vi "GV_FindEqualUnits.vi"(11 "TAGproperties":T1=[{"TAG"="ch0001", "Qtype"="PAQ", "TAGprop"={"Description"="", "EngUnits"="", "RangeH"=-1.0, "RangeL"=-1.0, "Resolution"=-1, "Obsolete"=FALSE, "ChangeDate"=timestamp(3692433115.085 s since 1904-01-01), "ChangeSource"="AVPP", "ChangeReason"="100 Unidentified TAGs sent by HISW", "TagFunc"=0}}, {"TAG"="ch0002", "Qtype"="PAQ", "TAGprop"={"Description"="", "EngUnits"="", "RangeH"=-1.0, "RangeL"=-1.0, "Resolution"=-1, "Obsolete"=FALSE, "ChangeDate"=timestamp(3692433115.085 s since 1904-01-01), "ChangeSource"="AVPP", "ChangeReason"="100 Unidentified TAGs sent by HISW", "TagFunc"=0}}, {"TAG"="ch0003", "Qtype"="PAQ", "TAGprop"={"Description"="", "EngUnits"="", "RangeH"=-1.0, "RangeL"=-1.0, "Resolution"=-1, "Obsolete"=FALSE, "ChangeDate"=timestamp(3692433115.085 s since 1904-01-01), "ChangeSource"="AVPP", "ChangeReason"="100 Unidentified TAGs sent by HISW", "TagFunc"=0}}, {"TAG"="ch0005", "Qtype"="PAQ", "TAGprop"={"Description"="", "EngUnits"="", "RangeH"=-1.0, "RangeL"=-1.0, "Resolution"=-1, "Obsolete"=FALSE, "ChangeDate"=timestamp(3692433115.085 s since 1904-01-01), "ChangeSource"="AVPP", "ChangeReason"="100 Unidentified TAGs sent by HISW", "TagFunc"=0}}, {"TAG"="ch0006", "Qtype"="PAQ", "TAGprop"={"Description"="", "EngUnits"="", "RangeH"=-1.0, "RangeL"=-1.0, "Resolution"=-1, "Obsolete"=FALSE, "ChangeDate"=timestamp(3692433115.085 s since 1904-01-01), "ChangeSource"="AVPP", "ChangeReason"="100 Unidentified TAGs sent by HISW", "TagFunc"=0}}] {"TAGprop"."TagFunc" format="%08x"; "TAGprop"."RangeL" format="%.2f"; "TAGprop"."RangeH" format="%.2f"}) -> (1 "TypeIdxPerTag":i32[](array[numeric]), 2 "IndexPerType":cluster{"EngUnit":string, "IdxPerType":i32[]}[](array[cluster]), 3 "EngUnitTypes":string[](array[string]))   [LabVIEW 2020, in "Sgraph_lib_V1.lvlib" / "Gviewer.lvclass"]
doc: "Andre Koelewijn, 17 aug 2021,\n\nSearch for identigal engineering units.\nThis VI delivers indexex to a list of equal engineering untis in case the Y-axis settings for every TAG needs to be made equal for every identical engeering unit type.\nThis is needed if the user want to compare graph values of several traces that have a similar engineering unit."
uses:
  Gviewer.lvclass
  DBAL/controls/DBAL_TAGprops.ctl
  DBAL/controls/DBAL_TAGpropEdit.ctl
  Common/controls/typedef_com_TagProp.ctl
  Builds/Sgraph_lib_V1.lvlib
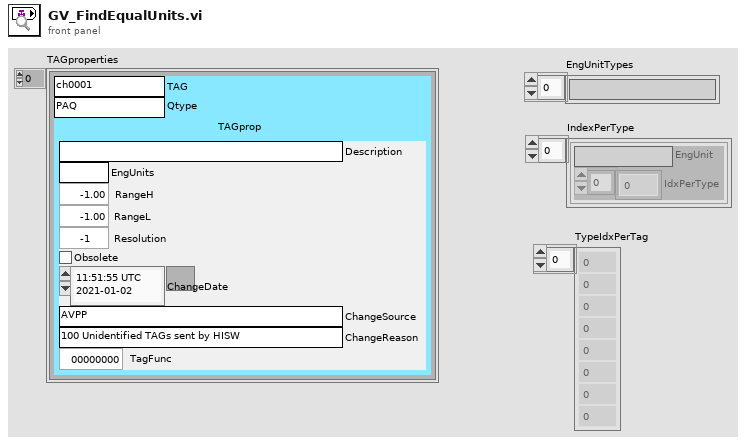
[diagram p1: front panel]
types:
  T1 = typedef "Sgraph_lib_V1.lvlib/DBAL_TAGprops.ctl" = T2[]
  T2 = typedef "Sgraph_lib_V1.lvlib/DBAL_TAGpropEdit.ctl" = cluster{"TAG":string, "Qtype":string, "TAGprop":T3}
  T3 = typedef "Sgraph_lib_V1.lvlib/typedef_com_TagProp.ctl" = cluster{"Description":string, "EngUnits":string, "RangeH":dbl, "RangeL":dbl, "Resolution":i32, "Obsolete":bool, "ChangeDate":timestamp, "ChangeSource":string, "ChangeReason":string, "TagFunc":u32}
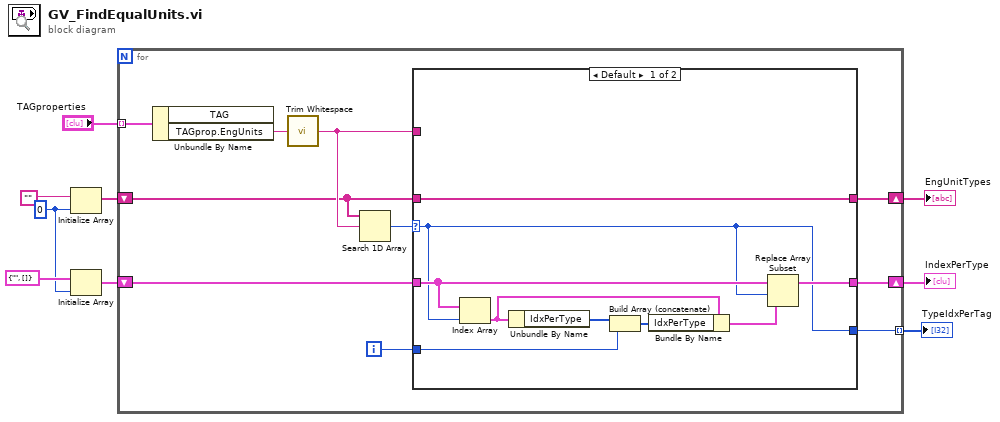
[diagram p0: block diagram]
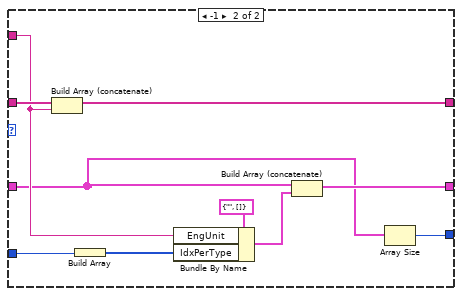
[diagram p2: hidden frame]
diagram:
  w4 = 0 ("dimension size")
  n1 = Initialize Array("", w4) -> (w7:string[])
  n2 = Initialize Array(cluster{"EngUnit":string, "IdxPerType":i32[]} {"EngUnit"="", "IdxPerType"=[]} ("IdxForOneType"), w4) -> (w3:cluster{"EngUnit":string, "IdxPerType":i32[]}[])
  n3 = for {
    tunnel: "TAGproperties" -> [w19] mode=indexing
    shift-right: [w14] -> w6
    shift-left: w7 -> [w15]
    shift-right: [w11] -> w2
    shift-left: w3 -> [w13]
    tunnel: [w10] -> w1 mode=indexing
    i -> [w12]
    n4 = Unbundle By Name(w19) -> ("TAGprop.EngUnits"=w18:string)  [unwired: 1 out]
    n5 = call <vilib>:"Trim Whitespace.vi"("string"=w18) -> ("trimmed string"=w16:string)  [unwired: 1 in]
    n6 = Search 1D Array(1D array=w15, element=w16) -> (index of element=w17:i32)  [unwired: 1 in]
    n7 = case shown="Default" w17 {
      selector: w17 -> [w20 _]
      tunnel: w16 -> [_ w34]
      tunnel: w15 -> [w28 w38]
      tunnel: [w28 w37] -> w14
      tunnel: w13 -> [w24 w30]
      tunnel: w12 -> [w21 w33]
      tunnel: [w22 w31] -> w11
      tunnel: [w20 w29] -> w10
      frame Default {
        n8 = Index Array(array=w24, index=w20) -> (element=w26:cluster{"EngUnit":string, "IdxPerType":i32[]})
        n9 = Unbundle By Name(w26) -> ("IdxPerType"=w27:i32[])
        n10 = Build Array (concatenate)(w27, w21) -> (w25:i32[])
        n11 = Bundle By Name(cluster=w26, "IdxPerType"=w25) -> (w23:cluster{"EngUnit":string, "IdxPerType":i32[]})
        n12 = Replace Array Subset(array=w24, new element=w23, index=w20) -> (w22:cluster{"EngUnit":string, "IdxPerType":i32[]}[])
      }
      frame -1 {
        n13 = Build Array (concatenate)(w38, w34) -> (w37:string[])
        n14 = Build Array(w33) -> (w32:i32[])
        n15 = Bundle By Name(cluster=cluster{"EngUnit":string, "IdxPerType":i32[]} {"EngUnit"="", "IdxPerType"=[]} ("IdxForOneType"), "EngUnit"=w34, "IdxPerType"=w32) -> (w35:cluster{"EngUnit":string, "IdxPerType":i32[]})
        n16 = Build Array (concatenate)(w30, w35) -> (w31:cluster{"EngUnit":string, "IdxPerType":i32[]}[])
        n17 = Array Size(array=w30) -> (size(s)=w29:i32)
      }
    }
  }
  "IndexPerType" <- w2
  "EngUnitTypes" <- w6
  "TypeIdxPerTag" <- w1
